vi "Clear Buffer.vi"(8 "error in (no error)":errorcluster, 11 "ONNX Class in":refnum<class "ONNX Class.lvclass">) -> (0 "error out":errorcluster, 3 "ONNX Class out":refnum<class "ONNX Class.lvclass">)   [LabVIEW 2017, in "ONNX Class Library.lvlib" / "ONNX Class.lvclass"]
uses:
  ONNX Class.lvclass
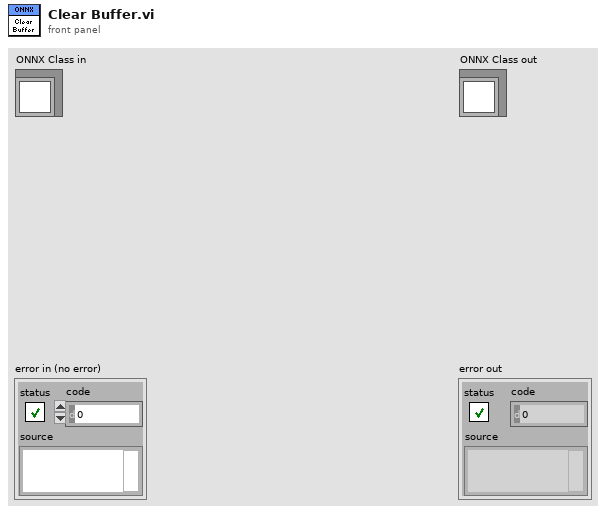
[diagram p1: front panel]
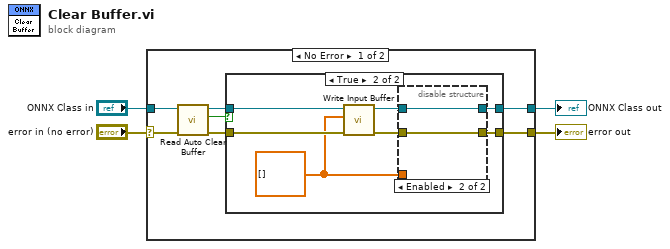
[diagram p0: block diagram]
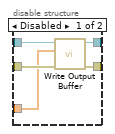
[diagram p3: hidden frame]
diagram:
  n1 = case shown="No Error" "error in (no error)" {
    selector: "error in (no error)" -> [w10 w29]
    tunnel: [w5 w29] -> w3
    tunnel: [w6 w28] -> w1
    tunnel: "ONNX Class in" -> [w11 w28]
    frame No Error {
      n2 = call-dynamic "Read Auto Clear Buffer.vi"("error in (no error)"=w10, "ONNX Class in"=w11) -> ("error out"=w7:errorcluster, "Auto Clear Buffer"=w9:bool, "ONNX Class out"=w8:refnum<class "ONNX Class.lvclass">)  [unwired: 7 in]
      n3 = case shown="True" w9 {
        tunnel: w8 -> [w13 w18]
        tunnel: w7 -> [w12 w17]
        tunnel: [w13 w20] -> w6
        tunnel: [w12 w19] -> w5
        frame False {
        }
        frame True {
          w14 = sgl[] [] ("initialized array")
          n4 = call-dynamic "Write Input Buffer.vi"("error in (no error)"=w17, "Input Buffer"=w14, "ONNX Class in"=w18) -> ("error out"=w15:errorcluster, "ONNX Class out"=w16:refnum<class "ONNX Class.lvclass">)  [unwired: 7 in]
          n5 = disable-structure shown="Enabled" {
            disable-tunnel: [w25 w27] -> w20
            disable-tunnel: [w24 w26] -> w19
            disable-tunnel: w16 -> [w23 w27]
            disable-tunnel: w15 -> [w22 w26]
            disable-tunnel: w14 -> [w21 _]
            frame Disabled {
              n6 = call-dynamic "Write Output Buffer.vi"("error in (no error)"=w22, "Output Buffer"=w21, "ONNX Class in"=w23) -> ("error out"=w24:errorcluster, "ONNX Class out"=w25:refnum<class "ONNX Class.lvclass">)  [unwired: 7 in]
            }
            frame Enabled {
            }
          }
        }
      }
    }
    frame Error {
    }
  }
  "error out" <- w3
  "ONNX Class out" <- w1
